vi "Color Interpolate CRI CQS table.vi"(4 "error in (no error)":errorcluster, 5 "a_tabelarray":dbl[](array[numeric]), 6 "a_CRI_CQSsample":u8, 7 "a_table":u8, 8 "a_NumInter":u16, 9 "a_data":dbl[](array[numeric])) -> (0 "error out":errorcluster, 1 "a_tabelarray out":dbl[](array[numeric]), 2 "function return":i16, 3 "a_data out":dbl[](array[numeric]))   [LabVIEW 2014, in "AvaSpec.lvlib" / "AVSirrad_support.lvlib" / "AVSirrad.lvlib"]
doc: "DLL_API short int __stdcall Color_GetColorRenderingIndex\n(\n DataType *a_data,\n unsigned char a_CIEResolution,\n unsigned char a_Observer,\n double *R_Values,\n double *CRI\n);"
uses:
  AVSirrad.lvlib
  AVSIRRAD/Examples/Labview/build/AVSirrad.dll
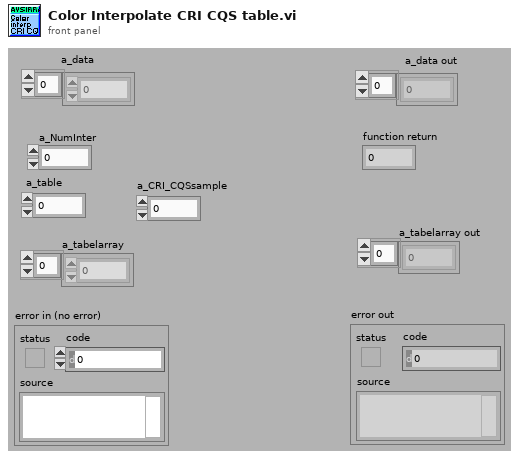
[diagram p1: front panel]
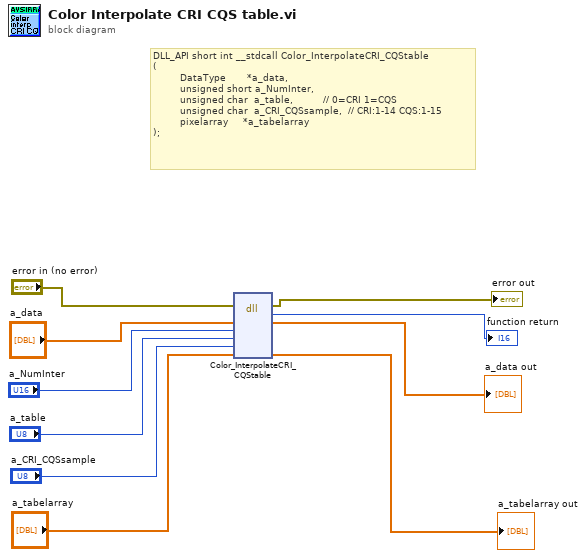
[diagram p0: block diagram]
diagram:
  # "DLL_API short int __stdcall Color_InterpolateCRI_CQStable\n(\n         DataType       *a_data,\n         unsigned short a_NumInter,\n         unsigned char  a_table,          // 0=CRI 1=CQS\n         unsigned char  a_CRI_CQSsample,  // CRI:1-14 CQS:1-15\n         pixelarray     *a_tabelarray\n);"
  n1 = dll-call lib="C:/AVSIRRAD/Examples/Labview/build/AVSirrad.*" fn="Color_InterpolateCRI_CQStable"(error in="error in (no error)", "a_data"="a_data", "a_NumInter"="a_NumInter", "a_table"="a_table", "a_CRI_CQSsample"="a_CRI_CQSsample", "a_tabelarray"="a_tabelarray") -> (error out=→"error out":errorcluster, "return type"=→"function return":i16, "a_data"=→"a_data out":dbl[], "a_tabelarray"=→"a_tabelarray out":dbl[])  [unwired: 5 in, 1 out]
